vi "工件信息输入_子VI.vi"(7 "Y Resolution":i32, 8 "X Resolution":i32, 9 "输入的灰度阈值":dbl) -> (0 "质量等级":string, 1 "模式选择":u16(ring) items=["只读穿透图", "穿透图和反射图结合"], 2 "灰度阈值":dbl, 3 "产品规格":cluster{"产品长度（周长）（mm）":dbl, "产品宽度（母线长）（mm）":dbl}, 4 "图像分辨率":T1)   [LabVIEW 2018]
panel:
  in  "模式选择（默认只读穿透图）":u16(ring) items=["只读穿透图", "穿透图和反射图结合"]
  in  "质量等级（请填入A/B/C，默认为B）":u16(ring) items=["A", "B", "C"]
  in  "灰度阈值（0-255）":dbl min=0.0 max=255.0 step=1.0 format="%#_13g"
  out "错误常量out":errorcluster
  in  "错误常量":errorcluster
  in  "停止按钮":bool
  in  "产品宽度（母线长）（mm）":dbl format="%#_13g"
  in  "产品长度（周长）（mm）":dbl format="%#_13g"
  in  "图像Y向分辨率（mm/像素）":dbl=1.0 format="%#_13g"
  in  "图像X向分辨率（mm/像素）":dbl=1.0 format="%#_13g"
  # "图像及工件参数输入"
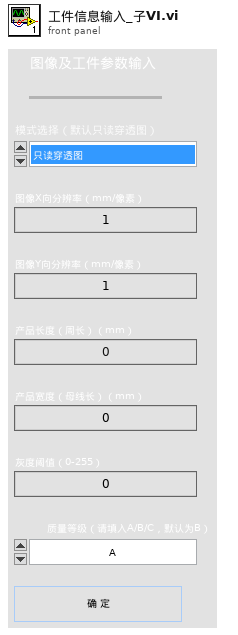
[diagram p1: front panel]
types:
  T1 = cluster{"图像X向分辨率（mm/像素）":dbl, "图像Y向分辨率（mm/像素）":dbl}
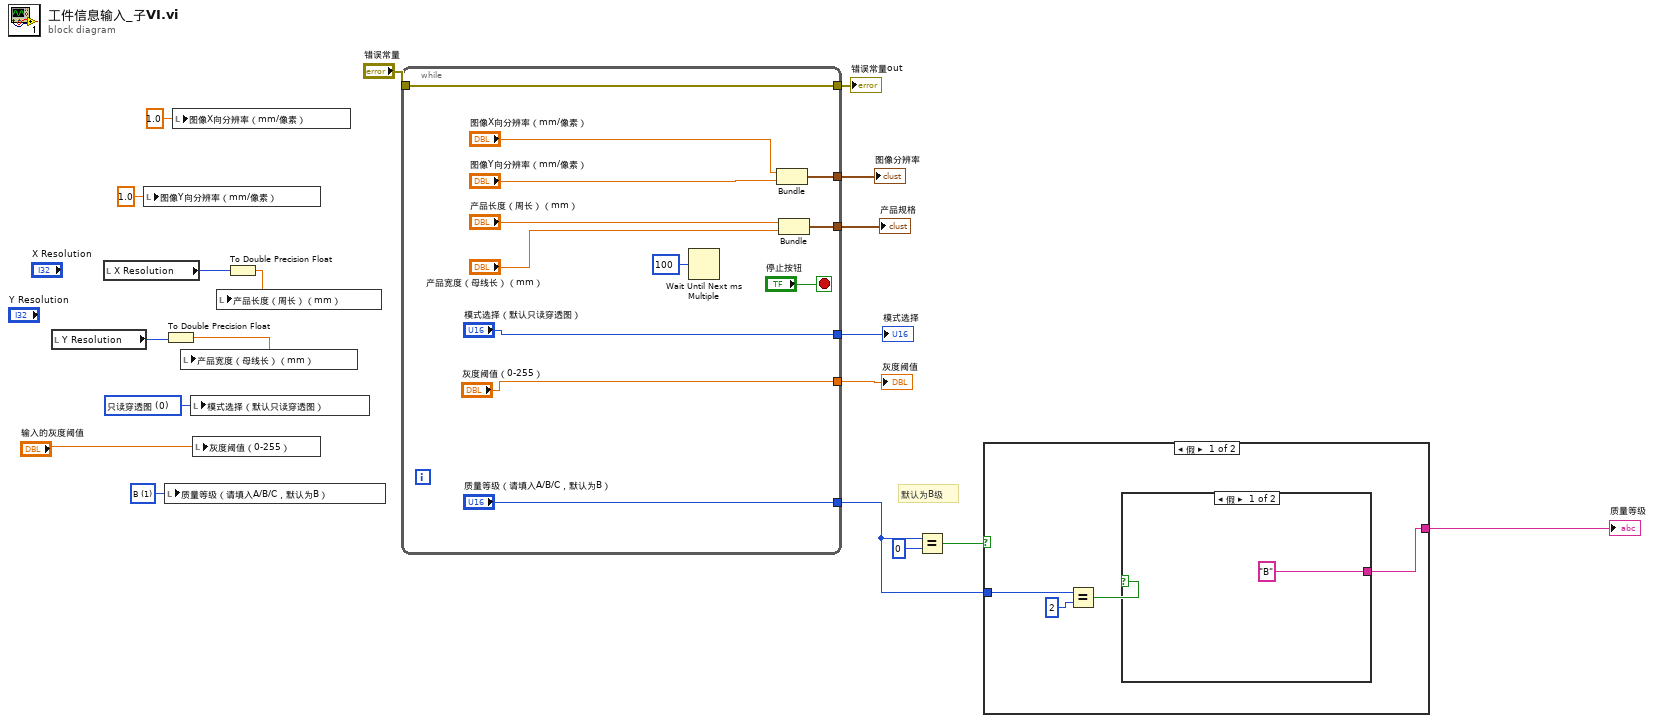
[diagram p0: block diagram]
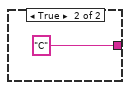
[diagram p2: hidden frame]
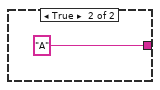
[diagram p3: hidden frame]
diagram:
  w12 = u16 1 items=["A", "B", "C"] ("质量等级（请填入A/B/C，默认为B）")
  w13 = u16 0 items=["只读穿透图", "穿透图和反射图结合"] ("模式选择（默认只读穿透图）")
  # "默认为B级"
  n1 = local read "Y Resolution"() -> (w5:i32)
  n2 = local read "X Resolution"() -> (w7:i32)
  n3 = local write "图像Y向分辨率（mm/像素）"(1.0 ("图像Y向分辨率（mm/像素）")) -> ()
  n4 = local write "质量等级（请填入A/B/C，默认为B）"(w12) -> ()
  n5 = To Double Precision Float(number=w5) -> (double precision float=w4:dbl)
  n6 = local write "图像X向分辨率（mm/像素）"(1.0 ("图像X向分辨率（mm/像素）")) -> ()
  n7 = local write "产品宽度（母线长）（mm）"(w4) -> ()
  n8 = local write "模式选择（默认只读穿透图）"(w13) -> ()
  n9 = local write "灰度阈值（0-255）"("输入的灰度阈值") -> ()
  n10 = To Double Precision Float(number=w7) -> (double precision float=w6:dbl)
  n11 = local write "产品长度（周长）（mm）"(w6) -> ()
  n12 = while {
    tunnel: [w31] -> w19
    tunnel: [w30] -> w18
    tunnel: "错误常量" -> [w24]
    tunnel: [w24] -> w16
    tunnel: ["灰度阈值（0-255）"] -> w15
    tunnel: ["质量等级（请填入A/B/C，默认为B）"] -> w8
    tunnel: ["模式选择（默认只读穿透图）"] -> w14
    stop <- "停止按钮" stop-if-true
    n13 = Wait Until Next ms Multiple(millisecond multiple=u32 100 ("毫秒倍数")) -> ()  [unwired: 1 out]
    n14 = Bundle("图像X向分辨率（mm/像素）"="图像X向分辨率（mm/像素）", "图像Y向分辨率（mm/像素）"="图像Y向分辨率（mm/像素）") -> (w31:T1)  [unwired: 1 in]
    n15 = Bundle("产品长度（周长）（mm）"="产品长度（周长）（mm）", "产品宽度（母线长）（mm）"="产品宽度（母线长）（mm）") -> (w30:cluster{"产品长度（周长）（mm）":dbl, "产品宽度（母线长）（mm）":dbl})  [unwired: 1 in]
  }
  "图像分辨率" <- w19
  "产品规格" <- w18
  "错误常量out" <- w16
  "灰度阈值" <- w15
  "模式选择" <- w14
  n16 = Equal?(x=w8, y=u16 0) -> (x = y?=w10:bool)
  n17 = case shown="假" w10 {
    tunnel: [w32 "A" ("质量等级")] -> w9
    tunnel: w8 -> [w34 _]
    frame False {
      n18 = Equal?(x=w34, y=u16 2) -> (x = y?=w33:bool)
      n19 = case shown="假" w33 {
        tunnel: ["B" ("质量等级") "C" ("质量等级")] -> w32
        frame False {
        }
        frame True {
        }
      }
    }
    frame True {
    }
  }
  "质量等级" <- w9
